vi "setColumn.vi"(8 "error in (no error)":errorcluster, 11 "reference in":refnum<class "excelFile.lvclass">) -> (0 "error out":errorcluster, 2 "column":i32, 3 "reference out":refnum<class "excelFile.lvclass">)   [LabVIEW 2014, in "excelFile.lvclass"]
uses:
  excelFile.lvclass
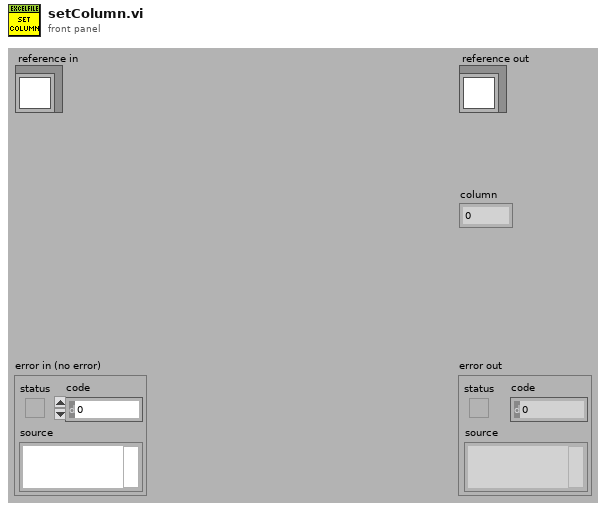
[diagram p1: front panel]
types:
  T1 = typedef "excelFile.lvclass/ObjectAttributesRef.ctl" = refnum<data-value>
  T2 = typedef "excelFile.lvclass/ObjectAttributes.ctl" = cluster{"MyAttribute":dbl, "path":string, "Refnum Excel":cluster{"Excel._Application":refnum<k7>, "Workbooks":refnum<k7>, "Open":refnum<k7>}, "data":string[][][], "save":bool, "fileType":T3, "rowsColor":u32[], "python_ref":refnum<class "python.lvclass">}
  T3 = typedef "excelFile.lvclass/fileType.ctl" = enum16{"devices", "items", "partsTracking"}
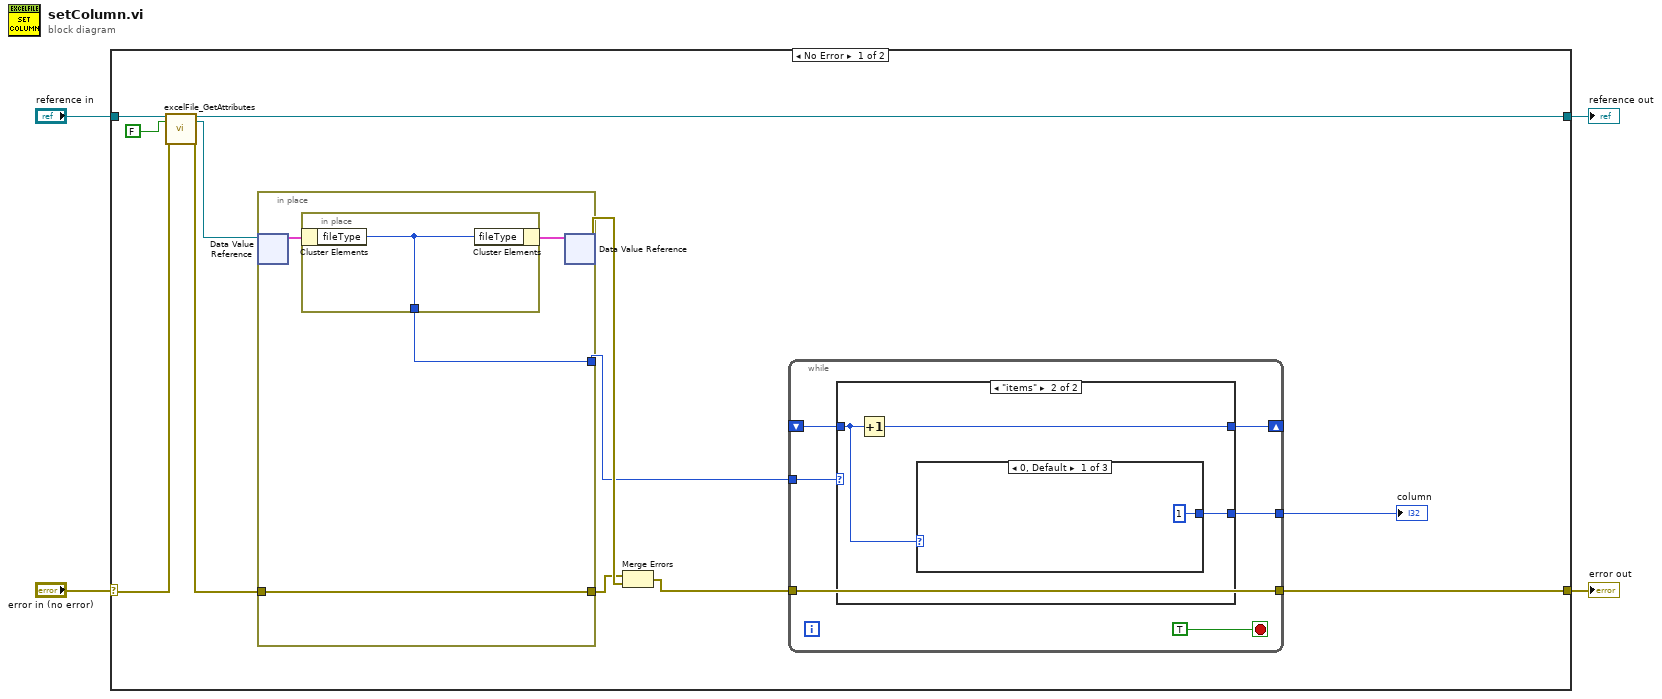
[diagram p0: block diagram]
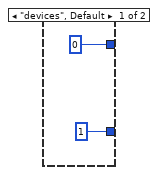
[diagram p2: hidden frame]
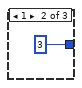
[diagram p3: hidden frame]
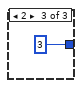
[diagram p4: hidden frame]
diagram:
  n1 = case shown="No Error" "error in (no error)" {
    selector: "error in (no error)" -> [w12 w37]
    tunnel: [w7 w37] -> w3
    tunnel: [w10 w36] -> w1
    tunnel: "reference in" -> [w14 w36]
    frame No Error {
      n2 = call "excelFile_GetAttributes.vi"("reference in"=w14, "return data? (T)"=FALSE, "error in (no error)"=w12) -> ("reference out"=w10:refnum<class "excelFile.lvclass">, "attributes ref"=w9:T1, "error out"=w11:errorcluster)  [unwired: 13 in, 1 out]
      n3 = in-place {
        in-place-border: w11 -> [w32]
        in-place-border: [w32] -> w15
        in-place-border: [w31] -> w5
        n4 = in-place-dvr #1(w9) -> (w33:T2)  [unwired: 1 out]
        n5 = in-place {
          in-place-border: [w35] -> w31
          n6 = in-place-cluster #2(w33) -> ("fileType"=w35:T3)
          n7 = in-place-cluster #2("fileType"=w35) -> (w34:T2)
        }
        n8 = in-place-dvr #1(w34) -> (w16:errorcluster)  [unwired: 1 out]
      }
      n9 = Merge Errors(w15, w16) -> (w8:errorcluster)
      n10 = while {
        tunnel: w8 -> [w22]
        tunnel: [w22] -> w7
        shift-right: [w20] -> _
        shift-left: _ -> [w19]
        tunnel: [w18] -> w6
        tunnel: w5 -> [w17]
        stop <- TRUE stop-if-true
        n11 = case shown="\"items\"" w17 {
          tunnel: [0 ("Column") w27] -> w20
          tunnel: w19 -> [_ w26]
          tunnel: [1 ("Column") w25] -> w18
          frame "devices", Default {
          }
          frame "items" {
            n12 = Increment(x=w26) -> (x+1=w27:i32)
            n13 = case shown="0, Default" w26 {
              tunnel: [1 ("Column") 3 ("Column") 3 ("Column")] -> w25
              frame 0, Default {
              }
              frame 1 {
              }
              frame 2 {
              }
            }
          }
        }
      }
      "column" <- w6
    }
    frame Error {
    }
  }
  "error out" <- w3
  "reference out" <- w1
